vi "ADC_USB.vi"() -> ()   [LabVIEW 2011]
uses:
  LabViewDllNet/bin/Debug/LabViewDllNet.dll
  <vilib>/Analysis/NI_AALPro.lvlib
panel:
  in  "Bytes To Read":u32
  in  "errorCorrection":bool
  out "Frequency":dbl
  out "Amplitude":dbl
  in  "Масштаб точно":i32
  out "Specific Harmonic":dbl
  out "THD":dbl
  out "SINAD (dB)":dbl
  in  "Offset":i32=2065
  in  "Часова розгортка точно":i32
  out "Спектр сигналу":dbl[](graph)
  in  "Часова розгортка грубо":i32(knob) scale=1.0..524000.0
  in  "Масштаб Х":i32(knob)=262293 scale=10.0..524000.0
  in  "Зміщення":i32(knob) scale=0.0..262000.0
  in  "sizeOfBuffer":i32=524000
  out "Вхідний сигнал":i32[](graph)
  out "errorsNumber":i32
  out "Bytes Read 2":u32
  out "Bytes Waiting 2":u32
  in  "stop 2":bool
  out "Device Description":string
  in  "Device Index":u32
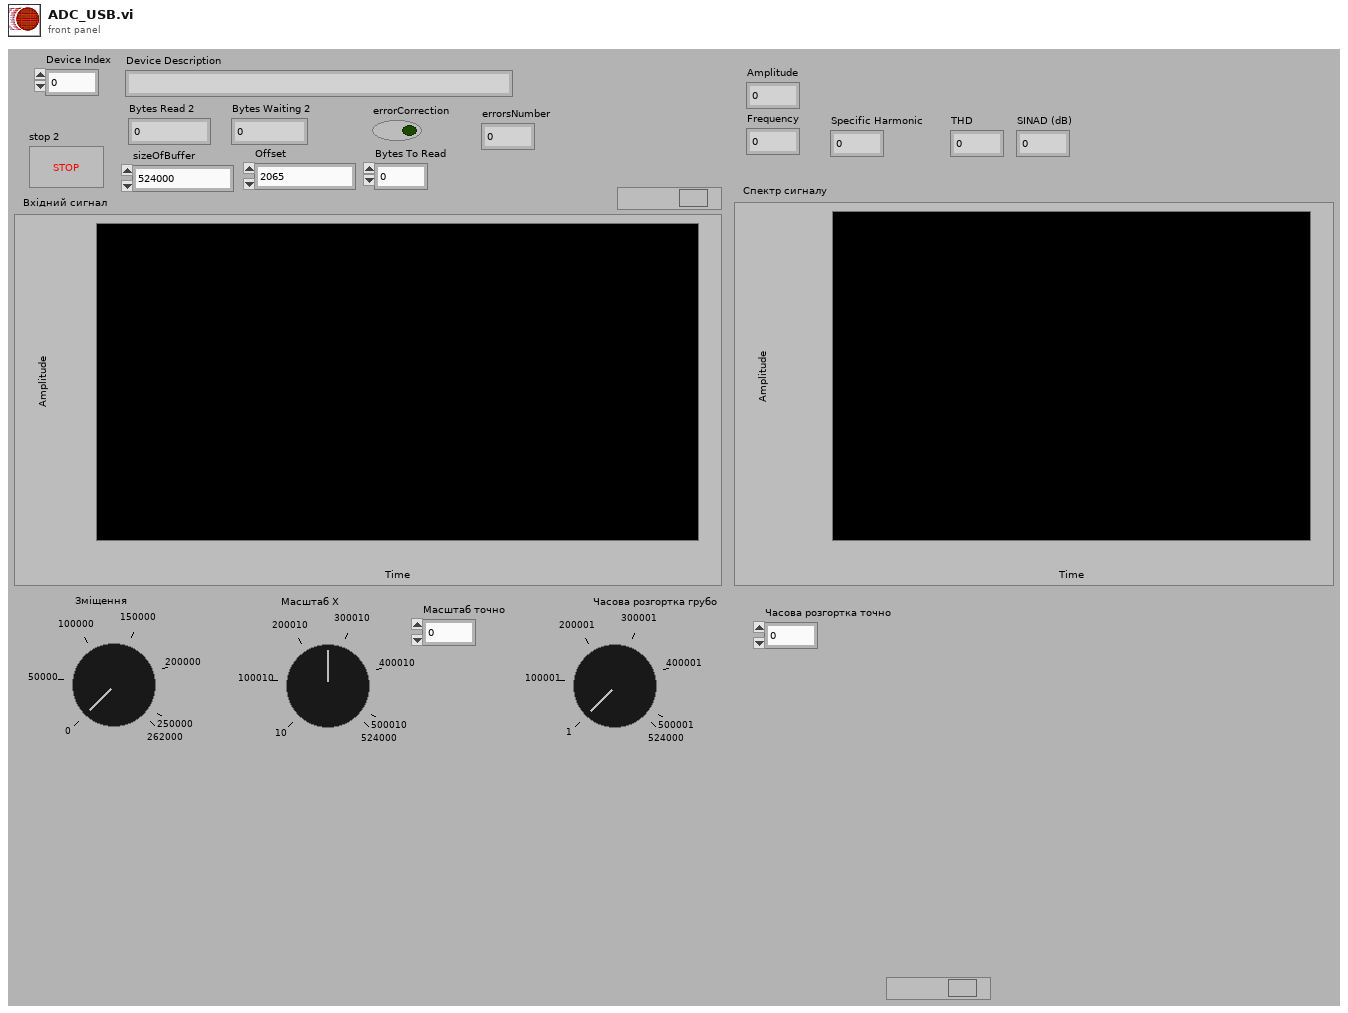
[diagram p1: front panel]
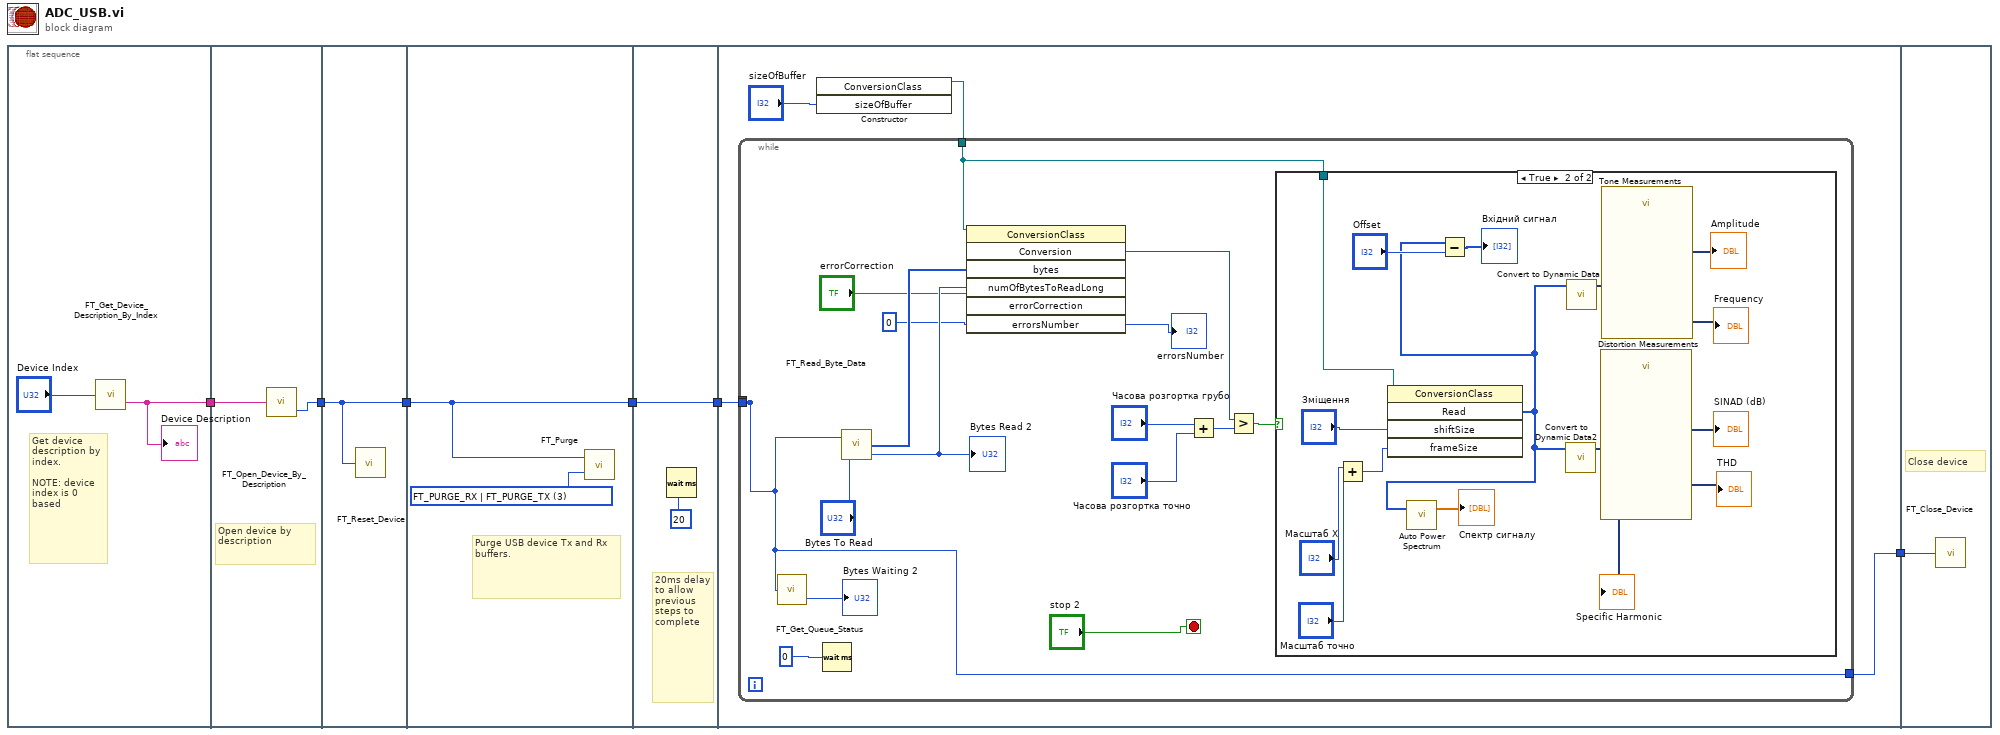
[diagram p0: block diagram]
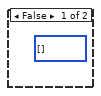
[diagram p2: hidden frame]
diagram:
  n1 = flat-sequence {
    tunnel: [w7] -> w1
    tunnel: [w10] -> w6
    tunnel: w1 -> [w9]
    tunnel: w6 -> [w11]
    tunnel: [w11] -> w4
    tunnel: [w12] -> w5
    tunnel: w4 -> [w12]
    tunnel: w5 -> [w14]
    tunnel: [w14] -> w2
    tunnel: [w16] -> w3
    tunnel: w2 -> [w19]
    tunnel: w3 -> [w52]
    frame #0 {
      # "Get device description by index.\n\nNOTE: device index is 0 based"
      n2 = call "FT_Get_Device_Description_By_Index.vi"("Device Index"="Device Index") -> ("Device Description"=w7:string)  [unwired: 1 out]
      "Device Description" <- w7
    }
    frame #1 {
      # "Open device by description"
      n3 = call "FT_Open_Device_By_Description.vi"("Device Description"=w9) -> ("Handle"=w10:u32)  [unwired: 1 out]
    }
    frame #2 {
      n4 = call "FT_Reset_Device.vi"("Handle"=w11) -> ()  [unwired: 1 out]
    }
    frame #3 {
      w13 = u32 3 items=["FT_PURGE_RX"=1, "FT_PURGE_TX"=2, "FT_PURGE_RX | FT_PURGE_TX"=3] ("Purge Flags")
      # "Purge USB device Tx and Rx  buffers."
      n5 = call "FT_Purge.vi"("Purge Flags"=w13, "Handle"=w12) -> ()  [unwired: 1 out]
    }
    frame #4 {
      # "20ms delay to allow previous steps to complete"
      n6 = Wait (ms)(milliseconds to wait=u32 20) -> ()  [unwired: 1 out]
    }
    frame #5 {
      n7 = constructor class="ConversionClass"("sizeOfBuffer"="sizeOfBuffer") -> (reference out=w17:refnum<k24>)  [unwired: 3 in, 3 out]
      n8 = while {
        tunnel: [w25] -> _
        tunnel: w19 -> [w25]
        tunnel: w17 -> [w24]
        tunnel: [w25] -> w16
        stop <- "stop 2" stop-if-true
        n9 = call "FT_Get_Queue_Status.vi"("Handle"=w25) -> ("Bytes Waiting"=→"Bytes Waiting 2":u32)  [unwired: 1 out]
        n10 = Wait (ms)(milliseconds to wait=u32 0) -> ()  [unwired: 1 out]
        n11 = call "FT_Read_Byte_Data.vi"("Handle"=w25, "Bytes To Read"="Bytes To Read") -> ("Read Data"=w33:u8[], "Bytes Read"=w29:u32)  [unwired: 1 out]
        "Bytes Read 2" <- w29
        n12 = invoke class="ConversionClass" method="Conversion"(reference=w24, "bytes"=w33, "numOfBytesToReadLong"=w29, "errorCorrection"="errorCorrection", "errorsNumber"=0) -> ("Conversion"=w30:i32, "errorsNumber"=→"errorsNumber":i32)  [unwired: 2 in, 5 out]
        n13 = Add(x="Часова розгортка грубо", y="Часова розгортка точно") -> (x+y=w28:i32)
        n14 = Greater?(x=w30, y=w28) -> (0:w31:bool)
        n15 = case shown="True" w31 {
          tunnel: w24 -> [_ w51]
          frame False {
            (unwired) i32[] [] ("Read")
          }
          frame True {
            n16 = Add(x="Масштаб Х", y="Масштаб точно") -> (x+y=w40:i32)
            n17 = invoke class="ConversionClass" method="Read"(reference=w51, "shiftSize"="Зміщення", "frameSize"=w40) -> ("Read"=w39:i32[])  [unwired: 2 in, 4 out]
            n18 = call <vilib>:"Auto Power Spectrum.vi"("Signal (V)"=w39) -> ("Power Spectrum (V^2 rms)"=→"Спектр сигналу":dbl[])  [unwired: 1 in, 1 out]
            n19 = Subtract(x=w39, y="Offset") -> (x-y=→"Вхідний сигнал":i32[])
            n20 = call "Convert to Dynamic Data2"("Array"=w39) -> ("Dynamic Data Type"=w46:dynamicdata)  [unwired: 3 in]
            n21 = call "Convert to Dynamic Data"("Array"=w39) -> ("Dynamic Data Type"=w38:dynamicdata)  [unwired: 3 in]
            n22 = call "Distortion Measurements"("Signals"=w46) -> ("SINAD (dB)"=→"SINAD (dB)":dynamicdata, "Specific Harmonic"=→"Specific Harmonic":dynamicdata, "THD"=→"THD":dynamicdata)  [unwired: 7 in, 1 out]
            n23 = call "Tone Measurements"("Signals"=w38) -> ("Frequency"=→"Frequency":dynamicdata, "Amplitude"=→"Amplitude":dynamicdata)  [unwired: 8 in, 1 out]
          }
        }
      }
    }
    frame #6 {
      # "Close device"
      n24 = call "FT_Close_Device.vi"("Handle"=w52) -> ()  [unwired: 1 out]
    }
  }
